vi "log analysis_gps.vi"() -> ()   [LabVIEW 2018] (continued)
log_raw\tgps_raw\t#INSPVAXA,USB3,0,48.0,FINESTEERING,2107,283336.950,02008000,471d,15824;INS_ALIGNMENT_COMPLETE,INS_RTKFIXED,37.37118094970,126.72303018769,7.8089,22.3000,0.0850,-0.2634,-0.0148,-0.368097924,-0.496074380,279.888293307,0.4400,0.2962,0.5694,0.1129,0.0927,0.0780,0.0968,0.1018,4.9757,0f000001,0*6cd4e320\n\tsystem status\tnormal 2 27.900000 0 0\trobot status\t194.436821\t116.615164\t7.808900\t-0.368098\t-0.496074\t170.111707\t0.186000\t-0.001000\n\t\n15:41:59.4\tlog_raw\tgps_raw\t#INSPVAXA,USB3,0,49.0,FINESTEERING,2107,283337.450,02008000,471d,15824;INS_ALIGNMENT_COMPLETE,INS_RTKFIXED,37.37118121756,126.72302900978,7.8099,22.3000,0.0919,-0.3084,-0.0188,-0.391974632,-0.310525962,279.833764071,0.4417,0.2966,0.5697,0.1134,0.0928,0.0781,0.0968,0.1018,4.9771,0f000001,0*732111a1\n\tsystem status\tnormal 2 27.900000 0 0\trobot status\t194.332484\t116.644895\t7.809900\t-0.391975\t-0.310526\t170.166236\t0.295000\t-0.006000\n\t\n15:41:59.9\tlog_raw\tgps_raw\t#DUALANTENNAHEADINGA,USB3,0,49.0,FINESTEERING,2107,283337.900,02008000,d426,15824;SOL_COMPUTED,L1_FLOAT,-1.000000000,237.924728394,61.700553894,0.0,151.721710205,100.643135071,\"631T\",14,6,6,5,04,00,20,03*b8043138\n\tsystem status\tnormal 2 27.900000 0 0\trobot status\t194.188208\t116.682010\t7.809100\t-0.393675\t-0.455807\t169.961143\t0.305000\t-0.011000\n\t\n15:42:00.4\tlog_raw\tgps_raw\t#DUALANTENNAHEADINGA,USB3,0,50.0,FINESTEERING,2107,283338.400,02008000,d426,15824;SOL_COMPUTED,L1_FLOAT,-1.000000000,237.905731201,60.774238586,0.0,143.960494995,94.373596191,\"631T\",14,6,6,5,04,00,20,03*a8a19996\n\tsystem status\tnormal 2 27.900000 0 0\trobot status\t194.064091\t116.716627\t7.808800\t-0.362161\t-0.573077\t169.900508\t0.294000\t-0.016000\n\t\n15:42:00.9\tlog_raw\tgps_raw\t#INSPVAXA,USB3,0,50.0,FINESTEERING,2107,283338.950,02008000,471d,15824;INS_ALIGNMENT_COMPLETE,INS_RTKFIXED,37.37118224254,126.72302419522,7.8081,22.3000,0.0973,-0.2877,-0.0182,-0.386859897,-0.840656461,280.267328107,0.4433,0.2968,0.5700,0.1133,0.0930,0.0781,0.0968,0.1018,4.9781,0f000001,0*f46e19c3\n\tsystem status\tnormal 2 27.900000 0 0\trobot status\t193.906018\t116.758662\t7.808100\t-0.386860\t-0.840656\t169.732672\t0.299000\t0.000000\n\t\n15:42:01.4\tlog_raw\tgps_raw\t\tsystem status\tnormal 2 27.900000 0 0\trobot status\t193.784168\t116.791420\t7.807600\t-0.352725\t-0.814458\t169.669579\t0.302000\t0.004000\n\t\n15:42:01.9\tlog_raw\tgps_raw\t#INSPVAXA,USB3,0,47.5,FINESTEERING,2107,283339.950,02000000,471d,15824;INS_ALIGNMENT_COMPLETE,INS_RTKFIXED,37.37118290995,126.72302108241,7.8055,22.3000,0.1047,-0.2801,-0.0151,-0.377109239,-0.859566836,280.447677121,0.4440,0.2973,0.5704,0.1133,0.0931,0.0781,0.0968,0.1018,4.9788,0f000001,0*ab964f25\n\tsystem status\tnormal 2 27.900000 0 0\trobot status\t193.630290\t116.832740\t7.805500\t-0.377109\t-0.859567\t169.552323\t0.296000\t-0.003000\n\t\n15:42:02.4\tlog_raw\tgps_raw\t#INSPVAXA,USB3,0,49.5,FINESTEERING,2107,283340.450,02000000,471d,15824;INS_ALIGNMENT_COMPLETE,INS_RTKFIXED,37.37118325232,126.72301952699,7.8038,22.3000,0.1007,-0.2812,-0.0170,-0.234742930,-0.655419935,280.541349843,0.4439,0.2974,0.5704,0.1133,0.0930,0.0781,0.0969,0.1018,4.9791,0f000001,0*59bc90eb\n\tsystem status\tnormal 2 27.900000 0 0\trobot status\t193.492514\t116.870741\t7.803800\t-0.234743\t-0.655420\t169.458650\t0.296000\t0.000000\n\t\n15:42:02.9\tlog_raw\tgps_raw\t#DUALANTENNAHEADINGA,USB3,0,49.5,FINESTEERING,2107,283340.900,02000000,d426,15824;SOL_COMPUTED,NARROW_FLOAT,-1.000000000,267.637573242,68.984275818,0.0,360.000000000,180.000000000,\"631T\",17,6,6,5,04,00,20,03*859e1115\n\tsystem status\tnormal 2 27.900000 0 0\trobot status\t193.368439\t116.905280\t7.802100\t-0.193901\t-0.504218\t169.351476\t0.300000\t0.000000\n\t\n15:42:03.4\tlog_raw\tgps_raw\t\tsystem status\tnormal 2 27.900000 0 0\trobot status\t193.227996\t116.944657\t7.800900\t-0.263364\t-0.492554\t169.255828\t0.293000\t0.006000\n\t\n15:42:03.9\tlog_raw\tgps_raw\t#INSPVAXA,USB3,0,44.0,FINESTEERING,2107,283341.950,02000000,471d,15824;INS_ALIGNMENT_COMPLETE,INS_RTKFIXED,37.37118432229,126.72301480701,7.8000,22.3000,0.1087,-0.2890,-0.0241,-0.323004853,-0.539804569,280.777320682,0.4437,0.2973,0.5706,0.1133,0.0929,0.0781,0.0969,0.1018,4.9792,0f000001,0*d82bda2e\n\tsystem status\tnormal 2 27.900000 0 0\trobot status\t193.074425\t116.989501\t7.800000\t-0.323005\t-0.539805\t169.222679\t0.299000\t0.000000\n\t\n15:42:04.4\tlog_raw\tgps_raw\t#INSPVAXA,USB3,0,46.5,FINESTEERING,2107,283342.450,02000000,471d,15824;INS_ALIGNMENT_COMPLETE,INS_RTKFIXED,37.37118468084,126.72301322867,7.7994,22.3000,0.1106,-0.2869,-0.0271,-0.331140922,-0.546506458,280.773428519,0.4432,0.2972,0.5705,0.1132,0.0928,0.0781,0.0969,0.1018,4.9794,0f000001,0*c730c292\n\tsystem status\tnormal 2 27.900000 0 0\trobot status\t192.934619\t117.029298\t7.799400\t-0.331141\t-0.546506\t169.226571\t0.260000\t0.069000\n\t\n15:42:04.9\tlog_raw\tgps_raw\t#INSPVAXA,USB3,0,46.5,FINESTEERING,2107,283342.950,02000000,471d,15824;INS_ALIGNMENT_COMPLETE,INS_RTKFIXED,37.37118504719,126.72301165338,7.7988,22.3000,0.1101,-0.2944,-0.0310,-0.265542746,-0.516192724,280.711326295,0.4432,0.2972,0.5705,0.1132,0.0928,0.0781,0.0969,0.1018,4.9794,0f000001,0*2bc99236\n\tsystem status\tnormal 2 27.900000 0 0\trobot status\t192.795082\t117.069960\t7.798800\t-0.265543\t-0.516193\t169.288674\t0.255000\t0.075000\n\t\n15:42:05.4\tlog_raw\tgps_raw\t#INSPVAXA,USB3,0,46.0,FINESTEERING,2107,283343.450,02000000,471d,15824;INS_ALIGNMENT_COMPLETE,INS_RTKFIXED,37.37118540426,126.72301007829,7.7983,22.3000,0.1044,-0.2953,-0.0281,-0.322294329,-0.503749733,280.647452797,0.4438,0.2974,0.5709,0.1134,0.0929,0.0781,0.0970,0.1019,4.9802,0f000001,0*02b1cd5a\n\tsystem status\tnormal 2 27.900000 0 0\trobot status\t192.655563\t117.109593\t7.798300\t-0.322294\t-0.503750\t169.352547\t0.292000\t0.019000\n\t\n15:42:05.9\tlog_raw\tgps_raw\t#INSPVAXA,USB3,0,46.0,FINESTEERING,2107,283343.950,02000000,471d,15824;INS_ALIGNMENT_COMPLETE,INS_RTKFIXED,37.37118578208,126.72300848824,7.7969,22.3000,0.1004,-0.2946,-0.0156,-0.222818059,-0.457044494,280.483100024,0.4438,0.2974,0.5709,0.1134,0.0929,0.0781,0.0970,0.1019,4.9802,0f000001,0*af3033cd\n\tsystem status\tnormal 2 27.900000 0 0\trobot status\t192.514719\t117.151528\t7.796900\t-0.222818\t-0.457044\t169.516900\t0.286000\t0.025000\n\t\n15:42:06.4\tlog_raw\tgps_raw\t#INSPVAXA,USB3,0,45.0,FINESTEERING,2107,283344.450,02000000,471d,15824;INS_ALIGNMENT_COMPLETE,INS_RTKFIXED,37.37118614793,126.72300689991,7.7943,22.3000,0.0993,-0.2872,-0.0172,-0.186993521,-0.511161636,280.230119633,0.4441,0.2974,0.5711,0.1134,0.0928,0.0781,0.0970,0.1019,4.9812,0f000001,0*b466b7e8\n\tsystem status\tnormal 2 27.900000 0 0\trobot status\t192.374027\t117.192135\t7.794300\t-0.186994\t-0.511162\t169.769880\t0.317000\t-0.007000\n\t\n15:42:06.9\tlog_raw\tgps_raw\t#INSPVAXA,USB3,0,45.0,FINESTEERING,2107,283344.950,02000000,471d,15824;INS_ALIGNMENT_COMPLETE,INS_RTKFIXED,37.37118650785,126.72300530954,7.7912,22.3000,0.0978,-0.2991,-0.0150,-0.269374143,-0.498749475,279.993433962,0.4441,0.2974,0.5711,0.1134,0.0928,0.0781,0.0970,0.1019,4.9812,0f000001,0*f4f3a5d7\n\tsystem status\tnormal 2 27.800000 0 0\trobot status\t192.233155\t117.232084\t7.791200\t-0.269374\t-0.498749\t170.006566\t0.322000\t-0.018000\n\t\n15:42:07.4\tlog_raw\tgps_raw\t#INSPVAXA,USB3,0,49.0,FINESTEERING,2107,283345.450,02000000,471d,15824;INS_ALIGNMENT_COMPLETE,INS_RTKFIXED,37.37118684878,126.72300372907,7.7899,22.3000,0.0930,-0.2956,-0.0147,-0.404221578,-0.693160058,279.694670090,0.4438,0.2972,0.5711,0.1134,0.0928,0.0781,0.0970,0.1019,4.9825,0f000001,0*306daf1e\n\tsystem status\tnormal 2 27.900000 0 0\trobot status\t192.093160\t117.269925\t7.789900\t-0.404222\t-0.693160\t170.305330\t0.238000\t0.091000\n\t\n15:42:07.9\tlog_raw\tgps_raw\t#INSPVAXA,USB3,0,49.0,FINESTEERING,2107,283345.950,02000000,471d,15824;INS_ALIGNMENT_COMPLETE,INS_RTKFIXED,37.37118719722,126.72300213566,7.7889,22.3000,0.0945,-0.2844,-0.0103,-0.444285686,-0.741424301,279.319475907,0.4438,0.2972,0.5711,0.1134,0.0928,0.0781,0.0970,0.1019,4.9825,0f000001,0*d5c67081\n\tsystem status\tnormal 2 27.800000 0 0\trobot status\t191.952018\t117.308600\t7.788900\t-0.444286\t-0.741424\t170.680524\t0.336000\t-0.047000\n\t\n15:42:08.4\tlog_raw\tgps_raw\t#INSPVAXA,USB3,0,45.5,FINESTEERING,2107,283346.450,02000000,471d,15824;INS_ALIGNMENT_COMPLETE,INS_RTKFIXED,37.37118745204,126.72300097325,7.7876,22.3000,0.0956,-0.2876,-0.0148,-0.514894680,-0.480743758,278.986298177,0.4452,0.2974,0.5713,0.1136,0.0929,0.0781,0.0970,0.1019,4.9840,0f000001,0*955fd833\n\tsystem status\tnormal 2 27.800000 0 0\trobot status\t191.849054\t117.336883\t7.787600\t-0.514895\t-0.480744\t171.013702\t0.179000\t0.076000\n\t\n15:42:08.9\tlog_raw\tgps_raw\t#INSPVAXA,USB3,0,45.5,FINESTEERING,2107,283346.950,02000000,471d,15824;INS_ALIGNMENT_COMPLETE,INS_RTKFIXED,37.37118779202,126.72299929144,7.7854,22.3000,0.1003,-0.2796,-0.0183,-0.357856906,-0.723006737,278.633509270,0.4452,0.2974,0.5713,0.1136,0.0929,0.0781,0.0970,0.1019,4.9840,0f000001,0*7a9ec2a9\n\tsystem status\tnormal 2 27.800000 0 0\trobot status\t191.700082\t117.374619\t7.785400\t-0.357857\t-0.723007\t171.366491\t0.207000\t0.120000\n\t\n15:42:09.4\tlog_raw\tgps_raw\t#INSPVAXA,USB3,0,50.5,FINESTEERING,2107,283347.450,02000000,471d,15824;INS_ALIGNMENT_COMPLETE,INS_RTKFIXED,37.37118807403,126.72299804089,7.7866,22.3000,0.0443,0.0041,-0.0189,-0.283640975,-0.830626211,278.365442964,0.4458,0.2975,0.5714,0.1138,0.0929,0.0781,0.0970,0.1020,4.9856,0f000001,0*be2d3140\n\tsystem status\tnormal 2 27.900000 0 0\trobot status\t191.589310\t117.405921\t7.786600\t-0.283641\t-0.830626\t171.634557\t0.068000\t-0.179000\n\t\n15:42:09.9\tlog_raw\tgps_raw\t#INSPVAXA,USB3,0,50.5,FINESTEERING,2107,283347.950,02000000,471d,15824;INS_ALIGNMENT_COMPLETE,INS_RTKFIXED,37.37118820355,126.72299809172,7.7880,22.3000,0.0534,-0.0137,-0.0152,-0.361607249,-0.776179806,278.567052976,0.4458,0.2975,0.5714,0.1138,0.0929,0.0781,0.0970,0.1020,4.9856,0f000001,0*5163b365\n\tsystem status\tnormal 2 27.900000 0 0\trobot status\t191.593812\t117.420295\t7.788000\t-0.361607\t-0.776180\t171.432947\t0.000000\t0.000000\n\t\n15:42:10.4\tlog_raw\tgps_raw\t#INSPVAXA,USB3,0,46.0,FINESTEERING,2107,283348.450,02008000,471d,15824;INS_ALIGNMENT_COMPLETE,INS_RTKFIXED,37.37118828288,126.72299813022,7.7895,22.3000,0.0516,-0.0114,-0.0144,-0.362235207,-0.776289694,278.558218042,0.4461,0.2975,0.5714,0.1165,0.0930,0.0781,0.0970,0.1020,4.9871,0f000001,0*00d92e93\n\tsystem status\tnormal 2 27.900000 0 0\trobot status\t191.597223\t117.429100\t7.789500\t-0.362235\t-0.776290\t171.441782\t0.000000\t0.000000\n\t\n15:42:10.9\tlog_raw\tgps_raw\t#INSPVAXA,USB3,0,46.0,FINESTEERING,2107,283348.950,02008000,471d,15824;INS_ALIGNMENT_COMPLETE,INS_RTKFIXED,37.37118838277,126.72299797344,7.7907,22.3000,0.0830,-0.1936,-0.0090,-0.388787979,-0.629836380,278.403166075,0.4461,0.2975,0.5714,0.1165,0.0930,0.0781,0.0970,0.1020,4.9871,0f000001,0*b6b1c278\n\tsystem status\tnormal 2 27.900000 0 0\trobot status\t191.583335\t117.440186\t7.790700\t-0.388788\t-0.629836\t171.596834\t0.161000\t-0.002000\n\t\n15:42:11.4\tlog_raw\tgps_raw\t\tsystem status\tnormal 2 27.900000 0 0\trobot status\t191.430583\t117.468941\t7.792500\t-0.272939\t-0.884725\t171.604531\t0.181000\t0.140000\n\t\n15:42:11.9\tlog_raw\tgps_raw\t#INSPVAXA,USB3,0,51.0,FINESTEERING,2107,283349.950,02008000,471d,15824;INS_ALIGNMENT_COMPLETE,INS_RTKFIXED,37.37118888254,126.72299463414,7.7948,22.3000,0.0854,-0.2630,-0.0100,-0.254550899,-0.902565471,278.109588384,0.4487,0.2974,0.5715,0.1138,0.0929,0.0781,0.0970,0.1020,4.9866,0f000001,0*b96721fd\n\tsystem status\tnormal 2 27.900000 0 0\trobot status\t191.287546\t117.495660\t7.794800\t-0.254551\t-0.902565\t171.890412\t0.328000\t-0.043000\n\t\n15:42:12.4\tlog_raw\tgps_raw\t#INSPVAXA,USB3,0,41.5,FINESTEERING,2107,283350.450,02008000,471d,15824;INS_ALIGNMENT_COMPLETE,INS_RTKFIXED,37.37118910944,126.72299305983,7.7973,22.3000,0.0714,-0.2778,-0.0014,-0.407636090,-0.881408174,277.766499487,0.4482,0.2974,0.5716,0.1138,0.0929,0.0781,0.0970,0.1019,4.9868,0f000001,0*7810372a\n\tsystem status\tnormal 2 27.900000 0 0\trobot status\t191.148096\t117.520845\t7.797300\t-0.407636\t-0.881408\t172.233501\t0.277000\t0.027000\n\t\n15:42:12.9\tlog_raw\tgps_raw\t#INSPVAXA,USB3,0,41.5,FINESTEERING,2107,283350.950,02008000,471d,15824;INS_ALIGNMENT_COMPLETE,INS_RTKFIXED,37.37118933104,126.72299159852,7.7984,22.3000,0.0589,-0.1073,-0.0277,-0.435946238,-1.120100302,277.342852709,0.4482,0.2974,0.5716,0.1138,0.0929,0.0781,0.0970,0.1019,4.9868,0f000001,0*557f5e08\n\tsystem status\tnormal 2 27.800000 0 0\trobot status\t191.018655\t117.545442\t7.798400\t-0.435946\t-1.120100\t172.657147\t0.186000\t-0.016000\n\t\n15:42:13.4\tlog_raw\tgps_raw\t#INSPVAXA,USB3,0,48.0,FINESTEERING,2107,283351.450,02008000,471d,15824;INS_ALIGNMENT_COMPLETE,INS_RTKFIXED,37.37118950550,126.72299029919,7.8000,22.3000,0.0990,-0.3064,-0.0104,-0.387241001,-0.965797752,277.134534078,0.4477,0.2974,0.5716,0.1154,0.0930,0.0781,0.0969,0.1019,4.9873,0f000001,0*28a1b0a6\n\tsystem status\tnormal 2 27.800000 0 0\trobot status\t190.903563\t117.564807\t7.800000\t-0.387241\t-0.965798\t172.865466\t0.353000\t0.019000\n\t\n15:42:13.9\tlog_raw\tgps_raw\t#INSPVAXA,USB3,0,48.0,FINESTEERING,2107,283351.950,02008000,471d,15824;INS_ALIGNMENT_COMPLETE,INS_RTKFIXED,37.37118970728,126.72298879350,7.8009,22.3000,0.0887,-0.3141,-0.0094,-0.308827403,-0.793055656,276.866791764,0.4477,0.2974,0.5716,0.1154,0.0930,0.0781,0.0969,0.1019,4.9873,0f000001,0*432182b8\n\tsystem status\tnormal 2 27.900000 0 0\trobot status\t190.770191\t117.587205\t7.800900\t-0.308827\t-0.793056\t173.133208\t0.348000\t-0.041000\n\t\n15:42:14.4\tlog_raw\tgps_raw\t#INSPVAXA,USB3,0,46.5,FINESTEERING,2107,283352.450,02000000,471d,15824;INS_ALIGNMENT_COMPLETE,INS_RTKFIXED,37.37118992961,126.72298725377,7.8025,22.3000,0.0817,-0.2903,-0.0217,-0.165574678,-0.563955548,276.694478613,0.4493,0.2975,0.5717,0.1140,0.0929,0.0781,0.0969,0.1019,4.9857,0f000001,0*b4fa8a95\n\tsystem status\tnormal 2 27.800000 0 0\trobot status\t190.633805\t117.611883\t7.802500\t-0.165575\t-0.563956\t173.305521\t0.233000\t0.102000\n\t\n15:42:14.9\tlog_raw\tgps_raw\t#INSPVAXA,USB3,0,46.5,FINESTEERING,2107,283352.950,02000000,471d,15824;INS_ALIGNMENT_COMPLETE,INS_RTKFIXED,37.37119014973,126.72298564431,7.8034,22.3000,0.0887,-0.3034,-0.0088,-0.249749639,-0.735815642,276.497650420,0.4493,0.2975,0.5717,0.1140,0.0929,0.0781,0.0969,0.1019,4.9857,0f000001,0*88cde8fe\n\tsystem status\tnormal 2 27.900000 0 0\trobot status\t190.491241\t117.636316\t7.803400\t-0.249750\t-0.735816\t173.502350\t0.271000\t0.033000\n\t\n15:42:15.4\tlog_raw\tgps_raw\t#INSPVAXA,USB3,0,50.0,FINESTEERING,2107,283353.450,02000000,471d,15824;INS_ALIGNMENT_COMPLETE,INS_RTKFIXED,37.37119037224,126.72298404949,7.8038,22.3000,0.0917,-0.2972,-0.0093,-0.357553897,-0.873995960,276.406472875,0.4475,0.2975,0.5716,0.1142,0.0929,0.0781,0.0969,0.1019,4.9865,0f000001,0*353531bb\n\tsystem status\tnormal 2 27.900000 0 0\trobot status\t190.349975\t117.661015\t7.803800\t-0.357554\t-0.873996\t173.593527\t0.236000\t0.101000\n\t\n15:42:15.9\tlog_raw\tgps_raw\t#INSPVAXA,USB3,0,50.0,FINESTEERING,2107,283353.950,02000000,471d,15824;INS_ALIGNMENT_COMPLETE,INS_RTKFIXED,37.37119060721,126.72298249352,7.8036,22.3000,0.0817,-0.2975,-0.0112,-0.379231468,-0.836316691,276.368569220,0.4475,0.2975,0.5716,0.1142,0.0929,0.0781,0.0969,0.1019,4.9865,0f000001,0*a3181148\n\tsystem status\tnormal 2 27.900000 0 0\trobot status\t190.212149\t117.687096\t7.803600\t-0.379231\t-0.836317\t173.631431\t0.265000\t0.054000\n\t\n15:42:16.4\tlog_raw\tgps_raw\t#INSPVAXA,USB3,0,49.0,FINESTEERING,2107,283354.450,02000000,471d,15824;INS_ALIGNMENT_COMPLETE,INS_RTKFIXED,37.37119085006,126.72298091760,7.8035,22.3000,0.0864,-0.2917,-0.0131,-0.320651128,-0.949485542,276.343611990,0.4461,0.2976,0.5717,0.1143,0.0929,0.0781,0.0969,0.1019,4.9881,0f000001,0*475d9375\n\tsystem status\tnormal 2 27.900000 0 0\trobot status\t190.072557\t117.714052\t7.803500\t-0.320651\t-0.949486\t173.656388\t0.205000\t0.129000\n\t\n15:42:16.9\tlog_raw\tgps_raw\t#INSPVAXA,USB3,0,49.0,FINESTEERING,2107,283354.950,02000000,471d,15824;INS_ALIGNMENT_COMPLETE,INS_RTKFIXED,37.37119110500,126.72297932256,7.8027,22.3000,0.0855,-0.2854,-0.0076,-0.293840157,-0.898732844,276.355365665,0.4461,0.2976,0.5717,0.1143,0.0929,0.0781,0.0969,0.1019,4.9881,0f000001,0*d412aada\n\tsystem status\tnormal 2 27.900000 0 0\trobot status\t189.931271\t117.742349\t7.802700\t-0.293840\t-0.898733\t173.644634\t0.284000\t0.021000\n\t\n15:42:17.4\tlog_raw\tgps_raw\t#INSPVAXA,USB3,0,51.0,FINESTEERING,2107,283355.450,02000000,471d,15824;INS_ALIGNMENT_COMPLETE,INS_RTKFIXED,37.37119134712,126.72297778450,7.8025,22.3000,0.0859,-0.2925,-0.0070,-0.311679134,-0.669484708,276.428044465,0.4456,0.2977,0.5720,0.1141,0.0929,0.0782,0.0969,0.1019,4.9893,0f000001,0*f22ce517\n\tsystem status\tnormal 2 27.900000 0 0\trobot status\t189.795032\t117.769224\t7.802500\t-0.311679\t-0.669485\t173.571956\t0.290000\t0.009000\n\t\n15:42:17.9\tlog_raw\tgps_raw\t#INSPVAXA,USB3,0,51.0,FINESTEERING,2107,283355.950,02000000,471d,15824;INS_ALIGNMENT_COMPLETE,INS_RTKFIXED,37.37119155988,126.72297664236,7.8028,22.3000,0.0638,-0.2658,-0.0150,-0.345823760,-0.347677441,276.253809925,0.4456,0.2977,0.5720,0.1141,0.0929,0.0782,0.0969,0.1019,4.9893,0f000001,0*f6cf90f8\n\tsystem status\tnormal 2 27.900000 0 0\trobot status\t189.693863\t117.792840\t7.802800\t-0.345824\t-0.347677\t173.746190\t0.282000\t-0.178000\n\t\n15:42:18.4\tlog_raw\tgps_raw\t#INSPVAXA,USB3,0,48.0,FINESTEERING,2107,283356.450,02000000,471d,15824;INS_ALIGNMENT_COMPLETE,INS_RTKFIXED,37.37119183139,126.72297483094,7.8027,22.3000,0.0833,-0.2731,-0.0206,-0.190515377,-0.472405138,276.460349150,0.4456,0.2978,0.5721,0.1141,0.0929,0.0782,0.0969,0.1019,4.9902,0f000001,0*837c9760\n\tsystem status\tnormal 2 27.900000 0 0\trobot status\t189.533411\t117.822977\t7.802700\t-0.190515\t-0.472405\t173.539651\t0.291000\t0.005000\n\t\n15:42:18.9\tlog_raw\tgps_raw\t#INSPVAXA,USB3,0,48.0,FINESTEERING,2107,283356.950,02000000,471d,15824;INS_ALIGNMENT_COMPLETE,INS_RTKFIXED,37.37119206486,126.72297337689,7.8027,22.3000,0.0844,-0.3387,-0.0089,-0.224745369,-0.389441077,276.529400158,0.4456,0.2978,0.5721,0.1141,0.0929,0.0782,0.0969,0.1019,4.9902,0f000001,0*8d83a1f7\n\tsystem status\tnormal 2 27.900000 0 0\trobot status\t189.404613\t117.848891\t7.802700\t-0.224745\t-0.389441\t173.470600\t0.312000\t0.007000\n\t\n15:42:19.4\tlog_raw\tgps_raw\t\tsystem status\tnormal 2 27.900000 0 0\trobot status\t189.265571\t117.875704\t7.803600\t-0.332884\t-0.361759\t173.397987\t0.286000\t-0.013000\n\t\n15:42:19.9\tlog_raw\tgps_raw\t#INSPVAXA,USB3,0,50.5,FINESTEERING,2107,283357.950,02000000,471d,15824;INS_ALIGNMENT_COMPLETE,INS_RTKFIXED,37.37119257424,126.72297012404,7.8046,22.3000,0.0855,-0.3001,-0.0197,-0.382775819,-0.574174795,276.720517942,0.4449,0.2976,0.5721,0.1140,0.0929,0.0782,0.0969,0.1019,4.9910,0f000001,0*b9513c1f\n\tsystem status\tnormal 2 27.900000 0 0\trobot status\t189.116481\t117.905431\t7.804600\t-0.382776\t-0.574175\t173.279482\t0.312000\t0.002000\n\t\n15:42:20.4\tlog_raw\tgps_raw\t#INSPVAXA,USB3,0,52.0,FINESTEERING,2107,283358.450,02000000,471d,15824;INS_ALIGNMENT_COMPLETE,INS_RTKFIXED,37.37119284307,126.72296856952,7.8054,22.3000,0.0869,-0.3084,-0.0144,-0.231977358,-0.593220103,276.754254189,0.4446,0.2976,0.5721,0.1139,0.0929,0.0782,0.0969,0.1019,4.9917,0f000001,0*6afd1835\n\tsystem status\tnormal 2 27.900000 0 0\trobot status\t188.978784\t117.935270\t7.805400\t-0.231977\t-0.593220\t173.245746\t0.301000\t0.000000\n\t\n15:42:20.9\tlog_raw\tgps_raw\t\tsystem status\tnormal 2 27.900000 0 0\trobot status\t188.837078\t117.965995\t7.806600\t-0.137793\t-0.481778\t173.220804\t0.294000\t0.000000\n\t\n15:42:21.4\tlog_raw\tgps_raw\t\tsystem status\tnormal 2 27.900000 0 0\trobot status\t188.694163\t117.995561\t7.808700\t-0.049687\t-0.403102\t173.144820\t0.296000\t0.000000\n\t\n15:42:21.9\tlog_raw\tgps_raw\t\tsystem status\tnormal 2 27.900000 0 0\trobot status\t188.549129\t118.025711\t7.811100\t-0.001917\t-0.448314\t173.070775\t0.307000\t-0.002000\n\t\n15:42:22.4\tlog_raw\tgps_raw\t\tsystem status\tnormal 2 27.900000 0 0\trobot status\t188.421935\t118.052449\t7.811200\t0.090407\t-0.517561\t173.058737\t0.226000\t-0.065000\n\t\n15:42:22.9\tlog_raw\tgps_raw\t#INSPVAXA,USB3,0,52.0,FINESTEERING,2107,283360.950,02008000,471d,15824;INS_ALIGNMENT_COMPLETE,INS_RTKFIXED,37.37119413375,126.72296080222,7.8105,22.3000,0.0870,-0.3889,-0.0160,0.035751589,-0.478950637,276.922392689,0.4441,0.2974,0.5721,0.1137,0.0929,0.0782,0.0970,0.1020,4.9937,0f000001,0*c5f9a7d1\n\tsystem status\tnormal 2 27.900000 0 0\trobot status\t188.290770\t118.078531\t7.810500\t0.035752\t-0.478951\t173.077607\t0.347000\t0.008000\n\t\n15:42:23.4\tlog_raw\tgps_raw\t\tsystem status\tnormal 2 27.900000 0 0\trobot status\t188.158077\t118.105638\t7.809700\t-0.145962\t-0.412339\t173.117591\t0.296000\t-0.005000\n\t\n15:42:23.9\tlog_raw\tgps_raw\t#INSPVAXA,USB3,0,51.0,FINESTEERING,2107,283361.950,02008000,471d,15824;INS_ALIGNMENT_COMPLETE,INS_RTKFIXED,37.37119465571,126.72295762324,7.8089,22.3000,0.0624,-0.2772,-0.0071,-0.112500356,-0.370528410,276.848536432,0.4446,0.2976,0.5722,0.1140,0.0929,0.0782,0.0970,0.1020,4.9950,0f000001,0*34f57e0c\n\tsystem status\tnormal 2 27.900000 0 0\trobot status\t188.009181\t118.136467\t7.808900\t-0.112500\t-0.370528\t173.151464\t0.338000\t-0.082000\n\t\n15:42:24.4\tlog_raw\tgps_raw\t#INSPVAXA,USB3,0,53.0,FINESTEERING,2107,283362.450,02008000,471d,15824;INS_ALIGNMENT_COMPLETE,INS_RTKFIXED,37.37119492880,126.72295600057,7.8073,22.3000,0.0711,-0.2912,-0.0111,0.131468491,-0.238366748,276.764142698,0.4434,0.2974,0.5719,0.1137,0.0929,0.0782,0.0970,0.1020,4.9960,0f000001,0*e2075610\n\tsystem status\tnormal 2 27.900000 0 0\trobot status\t187.865447\t118.166779\t7.807300\t0.131468\t-0.238367\t173.235857\t0.291000\t0.020000\n\t\n15:42:24.9\tlog_raw\tgps_raw\t\tsystem status\tnormal 2 27.900000 0 0\trobot status\t187.722244\t118.196735\t7.804800\t0.275217\t-0.097281\t173.319891\t0.255000\t0.076000\n\t\n15:42:25.4\tlog_raw\tgps_raw\t\tsystem status\tnormal 2 27.800000 0 0\trobot status\t187.580635\t118.224722\t7.803800\t0.210987\t-0.157671\t173.488063\t0.292000\t0.011000\n\t\n15:42:25.9\tlog_raw\tgps_raw\t\tsystem status\tnormal 2 27.800000 0 0\trobot status\t187.435600\t118.252018\t7.802900\t-0.001959\t-0.190708\t173.691503\t0.361000\t-0.089000\n\t\n15:42:26.4\tlog_raw\tgps_raw\t\tsystem status\tnormal 2 27.800000 0 0\trobot status\t187.292336\t118.279257\t7.803100\t0.128222\t-0.282878\t173.947517\t0.236000\t0.087000\n\t\n15:42:26.9\tlog_raw\tgps_raw\t#INSPVAXA,USB3,0,45.0,FINESTEERING,2107,283364.950,02000000,471d,15824;INS_ALIGNMENT_COMPLETE,INS_RTKFIXED,37.37119619456,126.72294796893,7.8017,22.3000,0.0616,-0.1768,-0.0159,0.378567506,-0.650059405,275.727416770,0.4438,0.2972,0.5717,0.1136,0.0929,0.0781,0.0970,0.1020,4.9990,0f000001,0*15cf5224\n\tsystem status\tnormal 2 27.800000 0 0\trobot status\t187.154018\t118.307275\t7.801700\t0.378568\t-0.650059\t174.272583\t0.151000\t0.051000\n\t\n15:42:27.4\tlog_raw\tgps_raw\t#INSPVAXA,USB3,0,50.0,FINESTEERING,2107,283365.450,02000000,471d,15824;INS_ALIGNMENT_COMPLETE,INS_RTKFIXED,37.37119642630,126.72294649498,7.8002,22.3000,0.0766,-0.2890,-0.0198,0.558482347,-0.615220653,275.473809484,0.4435,0.2971,0.5716,0.1149,0.0929,0.0782,0.0970,0.1020,5.0004,0f000001,0*3ebc86c2\n\tsystem status\tnormal 2 27.800000 0 0\trobot status\t187.023458\t118.332997\t7.800200\t0.558482\t-0.615221\t174.526191\t0.426000\t-0.153000\n\t\n15:42:27.9\tlog_raw\tgps_raw\t#INSPVAXA,USB3,0,50.0,FINESTEERING,2107,283365.950,02000000,471d,15824;INS_ALIGNMENT_COMPLETE,INS_RTKFIXED,37.37119665174,126.72294494158,7.7990,22.3000,0.0716,-0.3103,-0.0171,0.492140051,-0.494452644,275.229300180,0.4435,0.2971,0.5716,0.1149,0.0929,0.0782,0.0970,0.1020,5.0004,0f000001,0*39471351\n\tsystem status\tnormal 2 27.800000 0 0\trobot status\t186.885860\t118.358021\t7.799000\t0.492140\t-0.494453\t174.770700\t0.265000\t0.086000\n\t\n15:42:28.4\tlog_raw\tgps_raw\t#INSPVAXA,USB3,0,50.0,FINESTEERING,2107,283366.450,02000000,471d,15824;INS_ALIGNMENT_COMPLETE,INS_RTKFIXED,37.37119686528,126.72294336052,7.7960,22.3000,0.0816,-0.3018,-0.0151,0.434319121,-0.533460520,274.921153499,0.4443,0.2970,0.5716,0.1134,0.0928,0.0781,0.0970,0.1019,5.0004,0f000001,0*50c9815e\n\tsystem status\tnormal 2 27.800000 0 0\trobot status\t186.745812\t118.381724\t7.796000\t0.434319\t-0.533461\t175.078847\t0.296000\t0.023000\n\t\n15:42:28.9\tlog_raw\tgps_raw\t#INSPVAXA,USB3,0,50.0,FINESTEERING,2107,283366.950,02000000,471d,15824;INS_ALIGNMENT_COMPLETE,INS_RTKFIXED,37.37119708745,126.72294176624,7.7921,22.3000,0.0872,-0.3063,-0.0184,0.501847827,-0.459662834,274.603339422,0.4443,0.2970,0.5716,0.1134,0.0928,0.0781,0.0970,0.1019,5.0004,0f000001,0*071e2a71\n\tsystem status\tnormal 2 27.800000 0 0\trobot status\t186.604594\t118.406384\t7.792100\t0.501848\t-0.459663\t175.396661\t0.247000\t0.099000\n\t\n15:42:29.4\tlog_raw\tgps_raw\t#INSPVAXA,USB3,0,51.5,FINESTEERING,2107,283367.450,02000000,471d,15824;INS_ALIGNMENT_COMPLETE,INS_RTKFIXED,37.37119730646,126.72294018823,7.7897,22.3000,0.0762,-0.3201,-0.0092,0.455189651,-0.424726107,274.340978604,0.4433,0.2970,0.5715,0.1134,0.0928,0.0781,0.0969,0.1019,5.0012,0f000001,0*e5f1ee66\n\tsystem status\tnormal 2 27.800000 0 0\trobot status\t186.464816\t118.430694\t7.789700\t0.455190\t-0.424726\t175.659021\t0.347000\t-0.056000\n\t\n15:42:29.9\tlog_raw\tgps_raw\t#INSPVAXA,USB3,0,51.5,FINESTEERING,2107,283367.950,02000000,471d,15824;INS_ALIGNMENT_COMPLETE,INS_RTKFIXED,37.37119753251,126.72293860969,7.7876,22.3000,0.0837,-0.3172,-0.0165,0.501901315,-0.449092823,274.123001325,0.4433,0.2970,0.5715,0.1134,0.0928,0.0781,0.0969,0.1019,5.0012,0f000001,0*973b3c7d\n\tsystem status\tnormal 2 27.800000 0 0\trobot status\t186.324992\t118.455785\t7.787600\t0.501901\t-0.449093\t175.876999\t0.258000\t0.068000\n\t\n15:42:30.4\tlog_raw\tgps_raw\t#INSPVAXA,USB3,0,52.0,FINESTEERING,2107,283368.450,02000000,471d,15824;INS_ALIGNMENT_COMPLETE,INS_RTKFIXED,37.37119773991,126.72293703252,7.7857,22.3000,0.0763,-0.3107,-0.0130,0.507599979,-0.527583312,273.978239871,0.4424,0.2970,0.5714,0.1134,0.0929,0.0781,0.0969,0.1019,5.0025,0f000001,0*0977dbed\n\tsystem status\tnormal 2 27.900000 0 0\trobot status\t186.185288\t118.478807\t7.785700\t0.507600\t-0.527583\t176.021760\t0.246000\t0.084000\n\t\n15:42:30.9\tlog_raw\tgps_raw\t#INSPVAXA,USB3,0,52.0,FINESTEERING,2107,283368.950,02000000,471d,15824;INS_ALIGNMENT_COMPLETE,INS_RTKFIXED,37.37119794751,126.72293547014,7.7834,22.3000,0.0774,-0.3055,-0.0096,0.435923288,-0.448613725,273.801043422,0.4424,0.2970,0.5714,0.1134,0.0929,0.0781,0.0969,0.1019,5.0025,0f000001,0*82a00475\n\tsystem status\tnormal 2 27.800000 0 0\trobot status\t186.046895\t118.501850\t7.783400\t0.435923\t-0.448614\t176.198957\t0.267000\t0.053000\n\t\n15:42:31.4\tlog_raw\tgps_raw\t#INSPVAXA,USB3,0,48.5,FINESTEERING,2107,283369.450,02000000,471d,15824;INS_ALIGNMENT_COMPLETE,INS_RTKFIXED,37.37119813318,126.72293389966,7.7815,22.3000,0.0767,-0.3032,-0.0244,0.361736458,-0.446611692,273.637411763,0.4418,0.2971,0.5713,0.1133,0.0928,0.0781,0.0969,0.1019,5.0040,0f000001,0*7557722f\n\tsystem status\tnormal 2 27.900000 0 0\trobot status\t185.907785\t118.522460\t7.781500\t0.361736\t-0.446612\t176.362588\t0.319000\t-0.020000\n\t\n15:42:31.9\tlog_raw\tgps_raw\t#INSPVAXA,USB3,0,48.5,FINESTEERING,2107,283369.950,02000000,471d,15824;INS_ALIGNMENT_COMPLETE,INS_RTKFIXED,37.37119830413,126.72293271861,7.7791,22.3000,0.0693,-0.3514,-0.0262,0.354676713,-0.290741223,273.403270579,0.4418,0.2971,0.5713,0.1133,0.0928,0.0781,0.0969,0.1019,5.0040,0f000001,0*dc07d898\n\tsystem status\tnormal 2 27.800000 0 0\trobot status\t185.803169\t118.541435\t7.779100\t0.354677\t-0.290741\t176.596729\t0.271000\t0.022000\n\t\n15:42:32.4\tlog_raw\tgps_raw\t#INSPVAXA,USB3,0,51.0,FINESTEERING,2107,283370.450,02000000,471d,15824;INS_ALIGNMENT_COMPLETE,INS_RTKFIXED,37.37119850662,126.72293105558,7.7771,22.3000,0.0595,-0.2759,-0.0122,0.499717871,-0.539639528,273.303930409,0.4416,0.2971,0.5713,0.1136,0.0928,0.0781,0.0969,0.1019,5.0055,0f000001,0*54bb0a79\n\tsystem status\tnormal 2 27.900000 0 0\trobot status\t185.655861\t118.563911\t7.777100\t0.499718\t-0.539640\t176.696070\t0.382000\t-0.167000\n\t\n15:42:32.9\tlog_raw\tgps_raw\t#INSPVAXA,USB3,0,51.0,FINESTEERING,2107,283370.950,02000000,471d,15824;INS_ALIGNMENT_COMPLETE,INS_RTKFIXED,37.37119870016,126.72292944010,7.7758,22.3000,0.0653,-0.2856,-0.0114,0.438696368,-0.681338677,273.167424084,0.4416,0.2971,0.5713,0.1136,0.0928,0.0781,0.0969,0.1019,5.0055,0f000001,0*647e7aec\n\tsystem status\tnormal 2 27.900000 0 0\trobot status\t185.512764\t118.585395\t7.775800\t0.438696\t-0.681339\t176.832576\t0.329000\t-0.064000\n\t\n15:42:33.4\tlog_raw\tgps_raw\t#INSPVAXA,USB3,0,49.5,FINESTEERING,2107,283371.450,02000000,471d,15824;INS_ALIGNMENT_COMPLETE,INS_RTKFIXED,37.37119889562,126.72292784230,7.7739,22.3000,0.0592,-0.2777,-0.0188,0.430914391,-0.804071772,273.160470511,0.4407,0.2971,0.5713,0.1133,0.0928,0.0781,0.0970,0.1019,5.0069,0f000001,0*7216170f\n\tsystem status\tnormal 2 27.900000 0 0\trobot status\t185.371234\t118.607091\t7.773900\t0.430914\t-0.804072\t176.839529\t0.230000\t0.075000\n\t\n15:42:33.9\tlog_raw\tgps_raw\t#INSPVAXA,USB3,0,49.5,FINESTEERING,2107,283371.950,02000000,471d,15824;INS_ALIGNMENT_COMPLETE,INS_RTKFIXED,37.37119909971,126.72292622305,7.7712,22.3000,0.0658,-0.2761,-0.0279,0.370330042,-0.824005995,273.116118143,0.4407,0.2971,0.5713,0.1133,0.0928,0.0781,0.0970,0.1019,5.0069,0f000001,0*a32c8b2e\n\tsystem status\tnormal 2 27.900000 0 0\trobot status\t185.227803\t118.629745\t7.771200\t0.370330\t-0.824006\t176.883882\t0.263000\t0.039000\n\t\n15:42:34.4\tlog_raw\tgps_raw\t#INSPVAXA,USB3,0,45.0,FINESTEERING,2107,283372.450,02008000,471d,15824;INS_ALIGNMENT_COMPLETE,INS_RTKFIXED,37.37119927896,126.72292465996,7.7702,22.3000,0.0660,-0.3016,-0.0255,0.364775106,-0.625908727,273.037477195,0.4411,0.2970,0.5714,0.1133,0.0928,0.0782,0.0970,0.1019,5.0085,0f000001,0*0beb0134\n\tsystem status\tnormal 2 27.900000 0 0\trobot status\t185.089347\t118.649642\t7.770200\t0.364775\t-0.625909\t176.962523\t0.355000\t-0.081000\n\t\n15:42:34.9\tlog_raw\tgps_raw\t#INSPVAXA,USB3,0,45.0,FINESTEERING,2107,283372.950,02008000,471d,15824;INS_ALIGNMENT_COMPLETE,INS_RTKFIXED,37.37119946128,126.72292307094,7.7690,22.3000,0.0748,-0.2983,-0.0240,0.262839225,-0.610161608,272.980185551,0.4411,0.2970,0.5714,0.1133,0.0928,0.0782,0.0970,0.1019,5.0085,0f000001,0*152c78c5\n\tsystem status\tnormal 2 27.900000 0 0\trobot status\t184.948595\t118.669880\t7.769000\t0.262839\t-0.610162\t177.019814\t0.243000\t0.079000\n\t\n15:42:35.4\tlog_raw\tgps_raw\t\tsystem status\tnormal 2 27.900000 0 0\trobot status\t184.806869\t118.689448\t7.767200\t0.260818\t-0.574469\t177.023214\t0.359000\t-0.096000\n\t\n15:42:35.9\tlog_raw\tgps_raw\t#INSPVAXA,USB3,0,43.5,FINESTEERING,2107,283373.950,02008000,471d,15824;INS_ALIGNMENT_COMPLETE,INS_RTKFIXED,37.37119982399,126.72291987146,7.7651,22.3000,0.0739,-0.3179,-0.0233,0.300302749,-0.690108533,272.938320429,0.4412,0.2969,0.5713,0.1133,0.0928,0.0782,0.0970,0.1019,5.0100,0f000001,0*993f6fee\n\tsystem status\tnormal 2 27.900000 0 0\trobot status\t184.665190\t118.710141\t7.765100\t0.300303\t-0.690109\t177.061680\t0.258000\t0.062000\n\t\n15:42:36.4\tlog_raw\tgps_raw\t#INSPVAXA,USB3,0,50.5,FINESTEERING,2107,283374.450,02008000,471d,15824;INS_ALIGNMENT_COMPLETE,INS_RTKFIXED,37.37119999209,126.72291839607,7.7668,22.3000,0.0594,-0.2174,-0.0147,0.364736898,-0.828751718,272.875534675,0.4410,0.2967,0.5712,0.1132,0.0928,0.0781,0.0969,0.1019,5.0114,0f000001,0*e047289e\n\tsystem status\tnormal 2 27.900000 0 0\trobot status\t184.534502\t118.728801\t7.766800\t0.364737\t-0.828752\t177.124465\t0.180000\t0.086000\n\t\n15:42:36.9\tlog_raw\tgps_raw\t\tsystem status\tnormal 2 27.900000 0 0\trobot status\t184.389083\t118.747925\t7.767900\t0.296244\t-0.921949\t177.095023\t0.359000\t-0.095000\n\t\n15:42:37.4\tlog_raw\tgps_raw\t\tsystem status\tnormal 2 27.900000 0 0\trobot status\t184.249431\t118.765002\t7.767800\t0.178940\t-0.996236\t177.083237\t0.307000\t0.023000\n\t\n15:42:37.9\tlog_raw\tgps_raw\t\tsystem status\tnormal 2 27.900000 0 0\trobot status\t184.113700\t118.783148\t7.767200\t0.202623\t-0.979831\t177.159004\t0.284000\t0.036000\n\t\n15:42:38.4\tlog_raw\tgps_raw\t\tsystem status\tnormal 2 27.900000 0 0\trobot status\t183.975055\t118.802026\t7.766100\t0.382511\t-0.972564\t177.197755\t0.246000\t0.077000\n\t\n15:42:38.9\tlog_raw\tgps_raw\t\tsystem status\tnormal 2 27.900000 0 0\trobot status\t183.833621\t118.820661\t7.764600\t0.376253\t-1.039218\t177.146963\t0.273000\t0.035000\n\t\n15:42:39.4\tlog_raw\tgps_raw\t#INSPVAXA,USB3,0,44.5,FINESTEERING,2107,283377.450,02000000,471d,15824;INS_ALIGNMENT_COMPLETE,INS_RTKFIXED,37.37120096948,126.72290890698,7.7646,22.3000,0.0650,-0.3099,-0.0265,0.285363327,-1.158258500,272.876132148,0.4400,0.2965,0.5712,0.1130,0.0929,0.0781,0.0969,0.1018,5.0148,0f000001,0*301623f0\n\tsystem status\tnormal 2 27.900000 0 0\trobot status\t183.693974\t118.837294\t7.764600\t0.285363\t-1.158259\t177.123868\t0.283000\t0.021000\n\t\n15:42:39.9\tlog_raw\tgps_raw\t\tsystem status\tnormal 2 27.900000 0 0\trobot status\t183.557899\t118.854532\t7.764900\t0.220671\t-1.211812\t177.147934\t0.265000\t0.049000\n\t\n15:42:40.4\tlog_raw\tgps_raw\t\tsystem status\tnormal 2 27.900000 0 0\trobot status\t183.419275\t118.871549\t7.763600\t0.237304\t-1.121573\t177.075837\t0.296000\t-0.016000\n\t\n15:42:40.9\tlog_raw\tgps_raw\t\tsystem status\tnormal 2 27.900000 0 0\trobot status\t183.279309\t118.888744\t7.761500\t0.190736\t-1.195584\t177.076579\t0.159000\t0.116000\n\t\n15:42:41.4\tlog_raw\tgps_raw\t\tsystem status\tnormal 2 27.900000 0 0\trobot status\t183.154389\t118.903528\t7.761200\t0.106390\t-1.188739\t177.017879\t0.338000\t-0.012000\n\t\n15:42:41.9\tlog_raw\tgps_raw\t\tsystem status\tnormal 2 27.900000 0 0\trobot status\t183.020461\t118.920474\t7.760800\t0.126606\t-1.132471\t177.011493\t0.275000\t-0.015000\n\t\n15:42:42.4\tlog_raw\tgps_raw\t#INSPVAXA,USB3,0,51.5,FINESTEERING,2107,283380.450,02000000,471d,15824;INS_ALIGNMENT_COMPLETE,INS_RTKFIXED,37.37120187255,126.72289967744,7.7619,22.3000,0.0618,-0.2860,-0.0148,0.133286693,-1.082116386,273.127550287,0.4398,0.2963,0.5712,0.1130,0.0928,0.0781,0.0968,0.1018,5.0173,0f000001,0*f1da128c\n\tsystem status\tnormal 2 27.900000 0 0\trobot status\t182.876437\t118.937539\t7.761900\t0.133287\t-1.082116\t176.872450\t0.298000\t-0.002000\n\t\n15:42:42.9\tlog_raw\tgps_raw\t\tsystem status\tnormal 2 27.900000 0 0\trobot status\t182.743536\t118.954831\t7.763400\t0.158810\t-1.176712\t176.796168\t0.307000\t-0.006000\n\t\n15:42:43.4\tlog_raw\tgps_raw\t\tsystem status\tnormal 2 27.900000 0 0\trobot status\t182.601600\t118.973570\t7.763500\t0.285093\t-1.239822\t176.714144\t0.292000\t0.000000\n\t\n15:42:43.9\tlog_raw\tgps_raw\t\tsystem status\tnormal 2 27.900000 0 0\trobot status\t182.457823\t118.992057\t7.762100\t0.232613\t-1.372805\t176.584485\t0.297000\t-0.006000\n\t\n15:42:44.4\tlog_raw\tgps_raw\t\tsystem status\tnormal 2 27.900000 0 0\trobot status\t182.323688\t119.009377\t7.762300\t0.074241\t-1.302096\t176.531081\t0.313000\t-0.008000\n\t\n15:42:44.9\tlog_raw\tgps_raw\t\tsystem status\tnormal 2 27.900000 0 0\trobot status\t182.180579\t119.027841\t7.761000\t-0.087108\t-1.388354\t176.445712\t0.296000\t0.001000\n\t\n15:42:45.4\tlog_raw\tgps_raw\t\tsystem status\tnormal 2 27.900000 0 0\trobot status\t182.037764\t119.047018\t7.759800\t-0.141649\t-1.444424\t176.277281\t0.283000\t0.017000\n\t\n15:42:45.9\tlog_raw\tgps_raw\t\tsystem status\tnormal 2 27.900000 0 0\trobot status\t181.923667\t119.064096\t7.759400\t-0.243923\t-1.103452\t176.270179\t0.296000\t-0.014000\n\t\n15:42:46.5\tlog_raw\tgps_raw\t\tsystem status\tnormal 2 27.900000 0 0\trobot status\t181.769513\t119.081861\t7.757700\t-0.735243\t-1.067172\t176.123507\t0.308000\t-0.016000\n\t\n15:42:46.9\tlog_raw\tgps_raw\t\tsystem status\tnormal 2 27.900000 0 0\trobot status\t181.644662\t119.100474\t7.760500\t-0.847447\t-0.517212\t176.101137\t0.309000\t0.007000\n\t\n15:42:47.5\tlog_raw\tgps_raw\t\tsystem status\tnormal 2 27.900000 0 0\trobot status\t181.490040\t119.118961\t7.760100\t-1.104270\t-0.103260\t175.997676\t0.296000\t0.000000\n\t\n15:42:48.0\tlog_raw\tgps_raw\t\tsystem status\tnormal 2 27.900000 0 0\trobot status\t181.367056\t119.137989\t7.761800\t-1.084078\t0.271811\t175.992858\t0.300000\t-0.005000\n\t\n15:42:48.5\tlog_raw\tgps_raw\t\tsystem status\tnormal 2 27.900000 0 0\trobot status\t181.210526\t119.158794\t7.763900\t-1.333017\t0.496117\t175.718147\t0.294000\t0.003000\n\t\n15:42:49.0\tlog_raw\tgps_raw\t\tsystem status\tnormal 2 27.900000 0 0\trobot status\t181.083870\t119.179450\t7.767600\t-1.334438\t0.865965\t175.807967\t0.302000\t-0.003000\n\t\n15:42:49.5\tlog_raw\tgps_raw\t\tsystem status\tnormal 2 27.900000 0 0\trobot status\t180.935467\t119.200617\t7.771400\t-1.441033\t0.855107\t175.599058\t0.302000\t0.001000\n\t\n15:42:50.0\tlog_raw\tgps_raw\t\tsystem status\tnormal 2 27.900000 0 0\trobot status\t180.796344\t119.224112\t7.776300\t-1.195920\t0.890148\t175.619701\t0.295000\t-0.007000\n\t\n15:42:50.5\tlog_raw\tgps_raw\t\tsystem status\tnormal 2 27.900000 0 0\trobot status\t180.661219\t119.247314\t7.781800\t-1.072815\t0.915105\t175.535098\t0.186000\t-0.033000\n\t\n15:42:51.0\tlog_raw\tgps_raw\t\tsystem status\tnormal 2 27.900000 0 0\trobot status\t180.547113\t119.266983\t7.786600\t-1.145747\t0.967251\t175.632416\t0.325000\t0.034000\n\t\n15:42:51.5\tlog_raw\tgps_raw\t\tsystem status\tnormal 2 27.900000 0 0\trobot status\t180.400243\t119.289618\t7.792200\t-1.264948\t0.875571\t175.493513\t0.285000\t-0.018000\n\t\n15:42:52.0\tlog_raw\tgps_raw\t\tsystem status\tnormal 2 27.900000 0 0\trobot status\t180.249606\t119.313613\t7.796900\t-1.255880\t0.809862\t175.385444\t0.298000\t0.001000\n\t\n15:42:52.5\tlog_raw\tgps_raw\t\tsystem status\tnormal 2 27.900000 0 0\trobot status\t180.108377\t119.337632\t7.803200\t-1.038208\t0.719993\t175.369666\t0.297000\t0.000000\n\t\n15:42:53.0\tlog_raw\tgps_raw\t\tsystem status\tnormal 2 27.900000 0 0\trobot status\t179.966137\t119.360651\t7.809400\t-1.029423\t0.676051\t175.312171\t0.296000\t-0.003000\n\t\n15:42:53.5\tlog_raw\tgps_raw\t\tsystem status\tnormal 2 27.900000 0 0\trobot status\t179.823785\t119.382998\t7.816300\t-1.093555\t0.658379\t175.273158\t0.299000\t0.000000\n\t\n15:42:54.0\tlog_raw\tgps_raw\t\tsystem status\tnormal 2 27.900000 0 0\trobot status\t179.677465\t119.407059\t7.822400\t-0.968231\t0.561568\t175.232427\t0.292000\t-0.004000\n\t\n15:42:54.5\tlog_raw\tgps_raw\t\tsystem status\tnormal 2 27.900000 0 0\trobot status\t179.532294\t119.430555\t7.826900\t-0.908245\t0.611796\t175.191348\t0.300000\t0.016000\n\t\n15:42:55.0\tlog_raw\tgps_raw\t\tsystem status\tnormal 2 27.900000 0 0\trobot status\t179.378564\t119.453986\t7.830800\t-0.987990\t0.601637\t175.402662\t0.324000\t-0.013000\n\t\n15:42:55.5\tlog_raw\tgps_raw\t#INSPVAXA,USB3,0,47.5,FINESTEERING,2107,283393.500,02000000,471d,15824;INS_ALIGNMENT_COMPLETE,INS_RTKFIXED,37.37120674691,126.72285844800,7.8363,22.3000,0.0562,-0.2735,-0.0060,-0.936766245,0.447139039,273.783760430,0.4461,0.2973,0.5726,0.1135,0.0929,0.0782,0.0967,0.1016,4.9878,0f000001,0*0929eb09\n\tsystem status\tnormal 2 27.700000 0 0\trobot status\t179.224400\t119.478597\t7.836300\t-0.936766\t0.447139\t176.216240\t0.264000\t0.096000\n\t\n15:42:56.0\tlog_raw\tgps_raw\t\tsystem status\tnormal 2 27.700000 0 0\trobot status\t179.098226\t119.498204\t7.841000\t-0.696467\t0.376253\t177.103291\t0.272000\t0.072000\n\t\n15:42:56.5\tlog_raw\tgps_raw\t\tsystem status\tnormal 2 27.700000 0 0\trobot status\t178.956810\t119.517843\t7.845000\t-0.424842\t0.372701\t178.172914\t0.288000\t0.041000\n\t\n15:42:57.0\tlog_raw\tgps_raw\t\tsystem status\tnormal 2 27.600000 0 0\trobot status\t178.812709\t119.533421\t7.848200\t-0.421624\t0.127640\t179.305331\t0.225000\t0.153000\n\t\n15:42:57.5\tlog_raw\tgps_raw\t\tsystem status\tnormal 2 27.600000 0 0\trobot status\t
